vi "repulsive-force.vi"(5 "influence radius":dbl=500.0 format="%#_13g", 7 "multiplier":dbl=1.0 format="%#_13g", 8 "obstacle pos":dbl[](array[numeric])=[338.0392150878906, -254.06089782714844] format="%#_13g", 9 "force-type":enum16{"repulsive", "attractive"}(ring), 11 "agent pos":dbl[](array[numeric])=[3750.471435546875, 295.0052490234375] format="%#_13g") -> (1 "magnitude":dbl, 3 "force":dbl[](array[numeric]))   [LabVIEW 2018]
panel:
  in  "max force":dbl=3.0 format="%#_13g"
  in  "min dist":dbl=130.0 format="%#_13g"
  in  "power":dbl=65000.0 format="%#_13g"
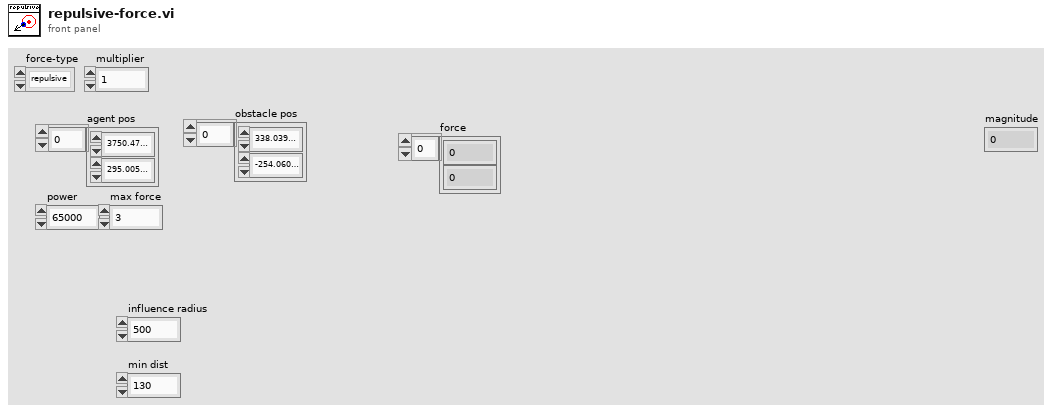
[diagram p1: front panel]
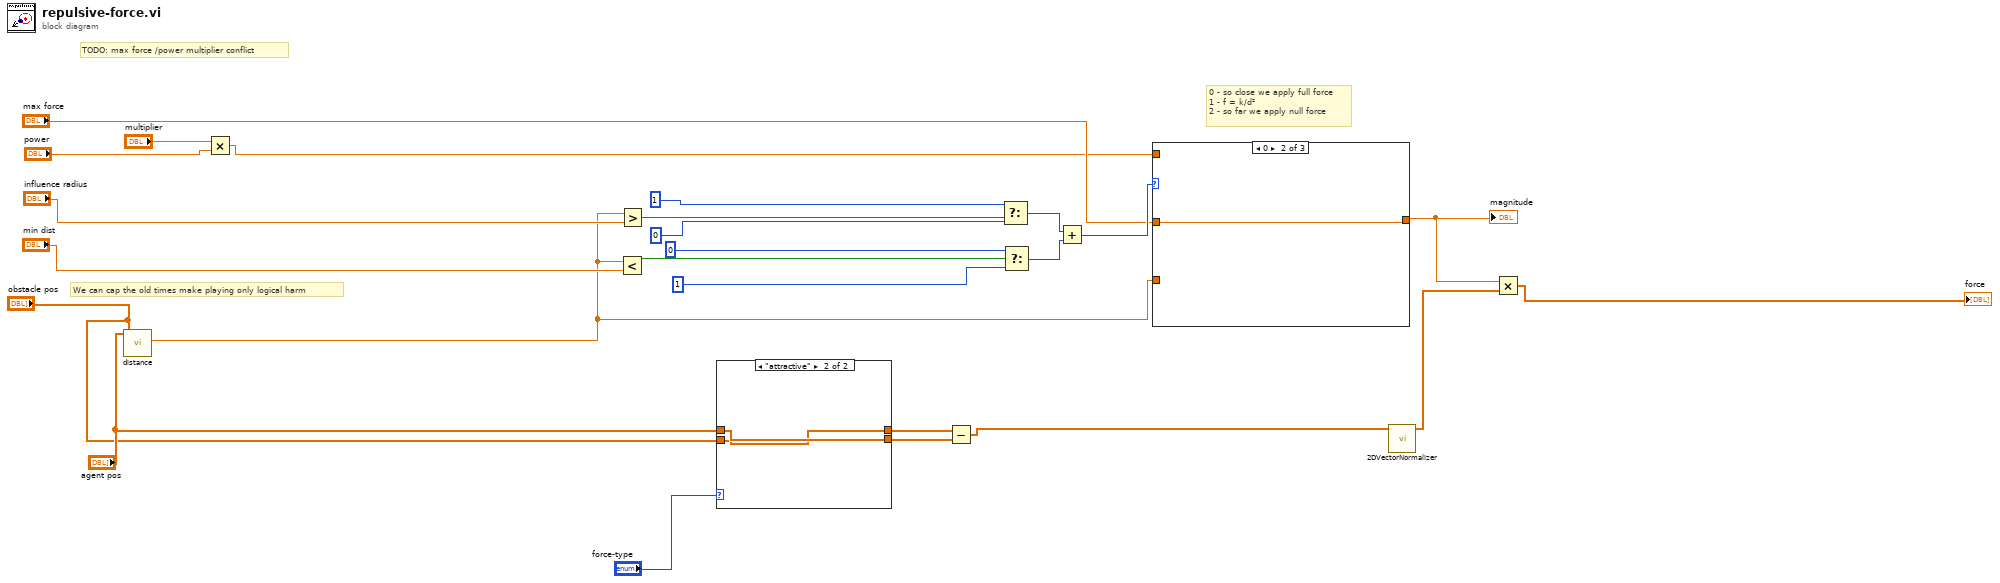
[diagram p0: block diagram]
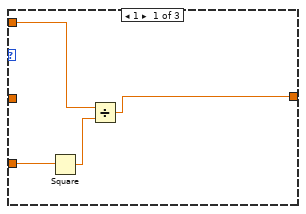
[diagram p3: hidden frame]
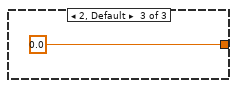
[diagram p4: hidden frame]
diagram:
  # "TODO: max force /power multiplier conflict"
  # "We can cap the old times make playing only logical harm"
  # "0 - so close we apply full force\n1 - f = k/d²\n2 - so far we apply null force"
  n1 = call "distance.vi"("target pos"="obstacle pos", "obj pos"="agent pos") -> ("sqrt(x)"=w14:dbl)  [unwired: 9 in]
  n2 = Multiply(x="multiplier", y="power") -> (x*y=w1:dbl)
  n3 = Less?(x=w14, y="min dist") -> (x < y?=w19:bool)
  n4 = Greater?(x=w14, y="influence radius") -> (0:w18:bool)
  n5 = case shown="\"attractive\"" "force-type" {
    tunnel: [w27 w28] -> w7
    tunnel: "agent pos" -> [w27 w29]
    tunnel: "obstacle pos" -> [w26 w28]
    tunnel: [w26 w29] -> w4
    frame "repulsive", Default {
    }
    frame "attractive" {
    }
  }
  n6 = Subtract(x=w7, y=w4) -> (x-y=w11:dbl[])
  n7 = Select(t=1, s=w18, f=0) -> (s? t:f=w17:i32)
  n8 = Select(t=0, s=w19, f=1) -> (s? t:f=w16:i32)
  n9 = Add(x=w17, y=w16) -> (x+y=w15:i32)
  n10 = case shown="0" w15 {
    tunnel: w14 -> [w33 _ _]
    tunnel: w1 -> [w31 _ _]
    tunnel: [w30 w34 0.0 ("max force")] -> w12
    tunnel: "max force" -> [_ w34 _]
    frame 1 {
      n11 = Square(x=w33) -> (x^2=w32:dbl)
      n12 = Divide(x=w31, y=w32) -> (x/y=w30:dbl)
    }
    frame 0 {
    }
    frame 2, Default {
    }
  }
  "magnitude" <- w12
  n13 = call "2DVectorNormalizer.vi"("2D vector"=w11) -> ("2D vector 2"=w10:dbl[])  [unwired: 10 in]
  n14 = Multiply(x=w12, y=w10) -> (x*y=→"force":dbl[])
